vi "onGenerateNewInboundChannel.vi"(8 "error in (no error)":errorcluster, 11 "Connection.NetworkStream in":refnum<class "Connection.NetworkStream.lvclass">) -> (0 "error out":errorcluster, 3 "Connection.NetworkStream out":refnum<class "Connection.NetworkStream.lvclass">)   [LabVIEW 2013, in "Connection.NetworkQueue_GOSPL.lvlib" / "Connection.NetworkStream.lvclass"]
uses:
  Connection.NetworkStream.lvclass
  Connection/Connection.lvclass
  Connection/Connection.lvclass/Connection.ctl
  <vilib>/LabVIEW Open Source Project/OpenURI/utilities/Extract URI Components.vi
  <vilib>/Utility/error.llb/Trim Whitespace.vi
  <vilib>/LabVIEW Open Source Project/Unicity/RandomStringGenerator/RandomStringGenerator.lvclass
  <vilib>/LabVIEW Open Source Project/OpenURI/openURI.lvlib
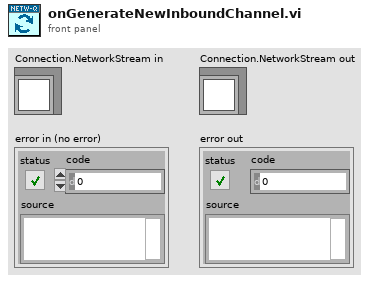
[diagram p1: front panel]
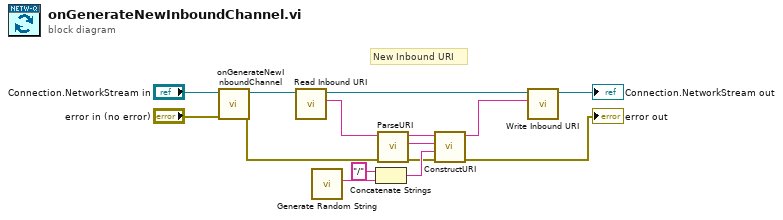
[diagram p0: block diagram]
diagram:
  # "New Inbound URI"
  n1 = call-parent "onGenerateNewInboundChannel.vi"("error in (no error)"="error in (no error)", "Connection in"="Connection.NetworkStream in") -> ("error out"=w2:errorcluster, "Connection out"=w4:refnum<class "Connection.NetworkStream.lvclass">)  [unwired: 8 in]
  n2 = call "Read Inbound URI.vi"("Connection in"=w4) -> ("Inbound URI"=w12:string, "Connection out"=w6:refnum<class "Connection.NetworkStream.lvclass">)  [unwired: 9 in]
  n3 = call <vilib>:"Generate Random String.vi"() -> ("Random String"=w7:string)  [unwired: 11 in]
  n4 = Concatenate Strings("/" ("string"), w7) -> (w11:string)
  n5 = call <vilib>:"ParseURI.vi"("error in"=w2, "URI"=w12) -> ("error out"=w5:errorcluster, "authority"=w10:string, "scheme"=w9:string)  [unwired: 4 in, 3 out]
  n6 = call <vilib>:"ConstructURI.vi"("error in"=w5, "path component"=w11, "authority"=w10, "scheme"=w9) -> ("error out"=→"error out":errorcluster, "URI"=w13:string)  [unwired: 6 in]
  n7 = call "Write Inbound URI.vi"("Inbound URI"=w13, "Connection in"=w6) -> ("Connection out"=→"Connection.NetworkStream out":refnum<class "Connection.NetworkStream.lvclass">)  [unwired: 9 in]
